vi "Polling.vi"() -> ()   [LabVIEW 2015]
panel:
  out "Time Stamp Control":timestamp
  in  "Time Check":bool
  out "Iteration":i32
  in  "Stop":bool
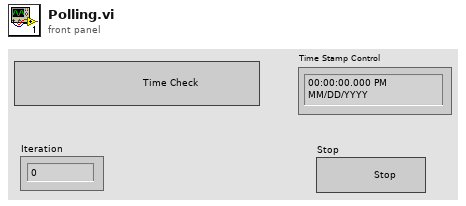
[diagram p1: front panel]
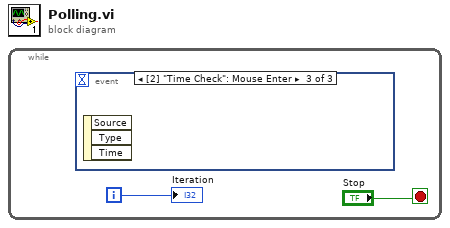
[diagram p0: block diagram]
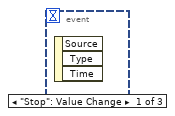
[diagram p2: hidden frame]
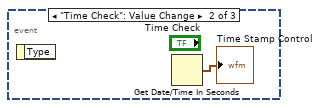
[diagram p3: hidden frame]
diagram:
  n1 = while {
    i -> [w2]
    stop <- "Stop" stop-if-true
    n2 = event shown="[2] \"Time Check\": Mouse Enter" {
      selector: _ -> [_ _ _]
      dyn-events: _ -> [_ _ _]
      timeout: _ -> [_ _ _]
      event "Stop": Value Change {
        n3 = event-data() -> ()  [unwired: 1 in, 3 out]
      }
      event "Time Check": Value Change {
        n4 = event-data() -> ()  [unwired: 1 in, 1 out]
        n5 = Get Date/Time In Seconds() -> (seconds since 1Jan1904=→"Time Stamp Control":timestamp)
      }
      event "Time Check": Mouse Enter {
        n6 = event-data() -> ()  [unwired: 1 in, 3 out]
      }
    }
    "Iteration" <- w2
  }
